vi "Draw(1).vi"(8 "error in (no error)":errorcluster, 10 "Picture in":picture, 11 "Ellipse in":refnum<class "Ellipse.lvclass">) -> (0 "error out":errorcluster, 2 "Picture out":picture, 3 "Ellipse out":refnum<class "Ellipse.lvclass">)   [LabVIEW 2015, in "Ellipse.lvclass"]
uses:
  Ellipse.lvclass
  Interfaces/Shape/Shape.lvclass/Shape.ctl
  Interfaces/Shape/Shape.lvclass
panel:
  # "NOTICE -- YOU MUST LEAVE THIS NOTICE IN PLACE.\n\nCopyright (c) 2017, LIANG LIU Shawn.Liu.cn@gmail.com\nAll rights reserved.\n\nRedistribution and use in source and binary forms, with or without modification, are permitted provided that the following conditions are met:\n-Redistributions of source code must retain the above copyright notice, this list of conditions and the following disclaimer.\n-Redistributions in binary form must reproduce the above copyright notice, this list of conditions and the following disclaimer in the documentation and/or other materials provided with the distribution.\n-Neither the name of the eLp nor the names of its contributors may be used to endorse or promote products derived from this software without specific prior written permission.\n\nTHIS SOFTWARE IS PROVIDED BY THE COPYRIGHT HOLDERS AND CONTRIBUTORS \"AS IS\" AND ANY EXPRESS OR IMPLIED WARRANTIES, INCLUDING, BUT NOT LIMITED TO, THE IMPLIED WARRANTIES OF MERCHANTABILITY AND FITNESS FOR A PARTICULAR PURPOSE ARE DISCLAIMED. IN NO EVENT SHALL THE COPYRIGHT HOLDER OR CONTRIBUTORS BE LIABLE FOR ANY DIRECT, INDIRECT, INCIDENTAL, SPECIAL, EXEMPLARY, OR CONSEQUENTIAL DAMAGES (INCLUDING, BUT NOT LIMITED TO, PROCUREMENT OF SUBSTITUTE GOODS OR SERVICES; LOSS OF USE, DATA, OR PROFITS; OR BUSINESS INTERRUPTION) HOWEVER CAUSED AND ON ANY THEORY OF LIABILITY, WHETHER IN CONTRACT, STRICT LIABILITY, OR TORT (INCLUDING NEGLIGENCE OR OTHERWISE) ARISING IN ANY WAY OUT OF THE USE OF THIS SOFTWARE, EVEN IF ADVISED OF THE POSSIBILITY OF SUCH DAMAGE."
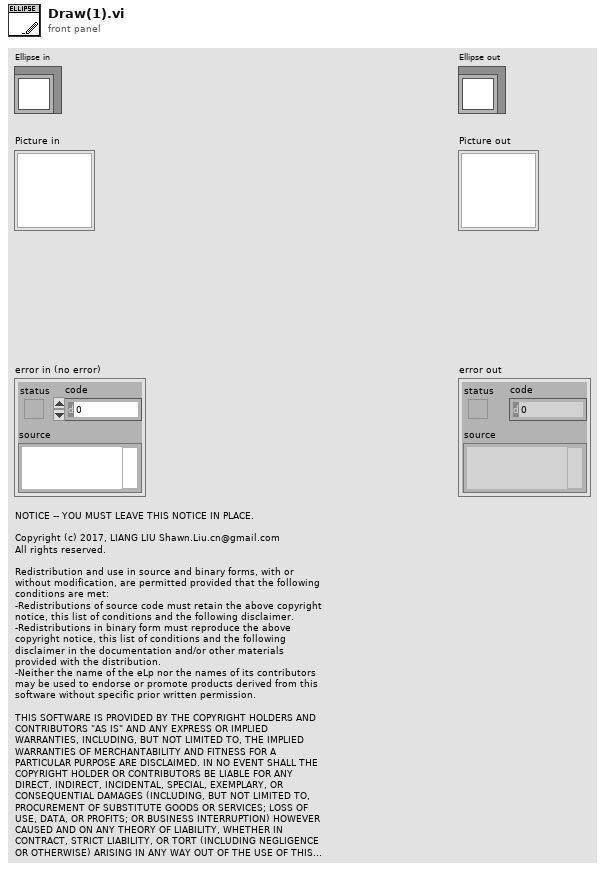
[diagram p1: front panel]
types:
  T1 = cluster{"left":i16, "top":i16, "right":i16, "bottom":i16}
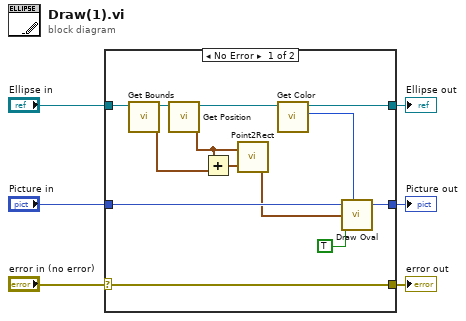
[diagram p0: block diagram]
diagram:
  n1 = case shown="No Error" "error in (no error)" {
    selector: "error in (no error)" -> [w19 w22]
    tunnel: "Ellipse in" -> [w18 w21]
    tunnel: [w15 w21] -> w2
    tunnel: "Picture in" -> [w11 w20]
    tunnel: [w10 w20] -> w1
    tunnel: [w19 w22] -> w4
    frame No Error {
      n2 = call "Get Bounds.vi"("Shape in"=w18) -> ("Bounds"=w14:cluster{"Width":u32, "Height":u32}, "Shape out"=w16:refnum<class "Ellipse.lvclass">)  [unwired: 9 in]
      n3 = call "Get Position.vi"("Shape in"=w16) -> ("Position"=w13:cluster{"Left":i32, "Top":i32}, "Shape out"=w17:refnum<class "Ellipse.lvclass">)  [unwired: 9 in]
      n4 = Add(x=w13, y=w14) -> (x+y=w12:cluster{u32, u32})
      n5 = call <vilib>:"Point2Rect.vi"("point b"=w12, "point a"=w13) -> ("rect"=w9:T1)
      n6 = call "Get Color.vi"("Shape in"=w17) -> ("Color"=w7:u32, "Shape out"=w15:refnum<class "Ellipse.lvclass">)  [unwired: 9 in]
      n7 = call <vilib>:"Draw Oval.vi"("picture"=w11, "rect"=w9, "fill?(F)"=TRUE, "color(black)"=w7) -> ("new picture"=w10:picture)  [unwired: 5 in]
    }
    frame Error {
    }
  }
  "error out" <- w4
  "Ellipse out" <- w2
  "Picture out" <- w1
